vi "LO M9347A.vi"(4 "Frequency GHz":dbl=1.0 format="%.10f", 5 "Exec":bool=TRUE, 6 "Enable":bool, 7 "Init":bool, 8 "error in (no error)":errorcluster, 9 "Power dBm":dbl format="%#.3f", 10 "Phase degree":dbl format="%#.4f", 11 "Chan":u16(ring)=1 items=["Channel 2"=2, "Channel 1"=1]) -> (0 "error out":errorcluster)   [LabVIEW 2023]
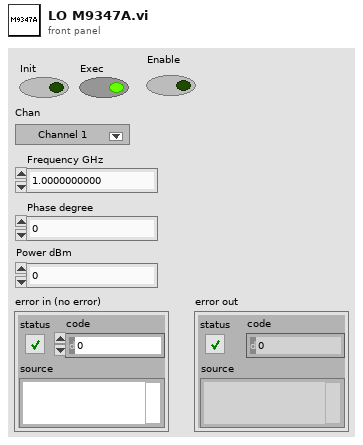
[diagram p1: front panel]
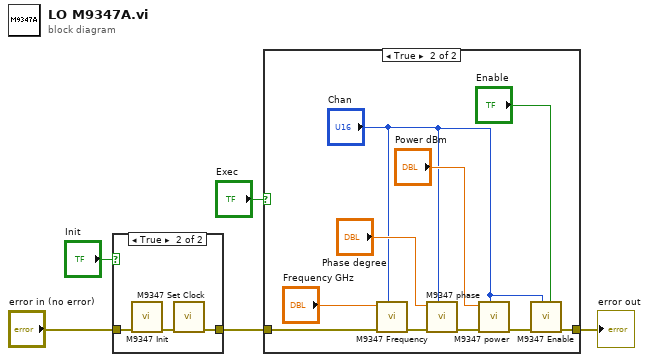
[diagram p0: block diagram]
diagram:
  n1 = case shown="True" "Init" {
    tunnel: "error in (no error)" -> [w6 w9]
    tunnel: [w6 w7] -> w2
    frame False {
    }
    frame True {
      n2 = call "M9347 Init.vi"("error in (no error)"=w9) -> ("error out"=w8:errorcluster)  [unwired: 10 in]
      n3 = call "M9347 Set Clock.vi"("error in (no error)"=w8) -> ("error out"=w7:errorcluster)  [unwired: 10 in]
    }
  }
  n4 = case shown="True" "Exec" {
    tunnel: w2 -> [w10 w20]
    tunnel: [w10 w13] -> w1
    frame False {
    }
    frame True {
      n5 = call "M9347 Frequency.vi"("Chan"="Chan", "error in (no error)"=w20, "Frequency GHz"="Frequency GHz") -> ("error out"=w19:errorcluster)  [unwired: 8 in]
      n6 = call "M9347 phase.vi"("Chan"="Chan", "error in (no error)"=w19, "Phase degree"="Phase degree") -> ("error out"=w18:errorcluster)  [unwired: 8 in]
      n7 = call "M9347 power.vi"("Chan"="Chan", "error in (no error)"=w18, "Power dBm"="Power dBm") -> ("error out"=w14:errorcluster)  [unwired: 8 in]
      n8 = call "M9347 Enable.vi"("Enable"="Enable", "Chan"="Chan", "error in (no error)"=w14) -> ("error out"=w13:errorcluster)  [unwired: 8 in]
    }
  }
  "error out" <- w1
